vi "RT Loop - Log Data_1.vi"(7 "G1 trigger":bool, 8 "error in (no error)":errorcluster, 9 "Log File out":refnum<k34>, 10 "Array":waveform(dbl)[](array[waveform]), 11 "Message Queue":refnum<queue>) -> ()   [LabVIEW 2017]
doc: "Receive triggered data from Analyze Acceleration Loop and log the data to disk."
uses:
  Globals/Global - All RT Loop Stop.vi
  UI Error Handlers/support/Message Queue/Message Cluster.ctl
  UI Error Handlers/support/Message Queue/Message Queue.lvlib
panel:
  out "AVI Path":path
  out "Acceleration Log Folder":path=path "/home/lvuser/Log/logfiles_deploy"
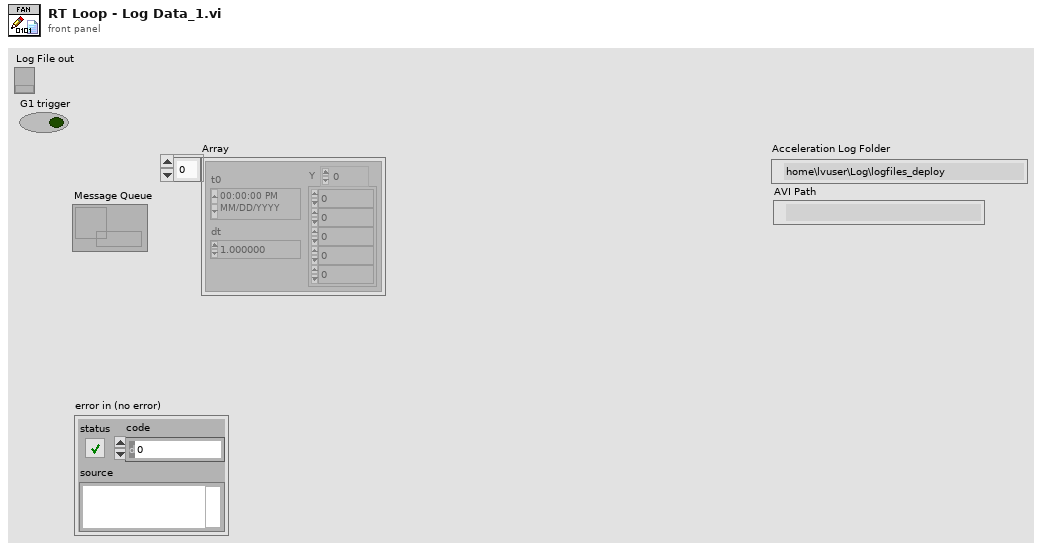
[diagram p1: front panel]
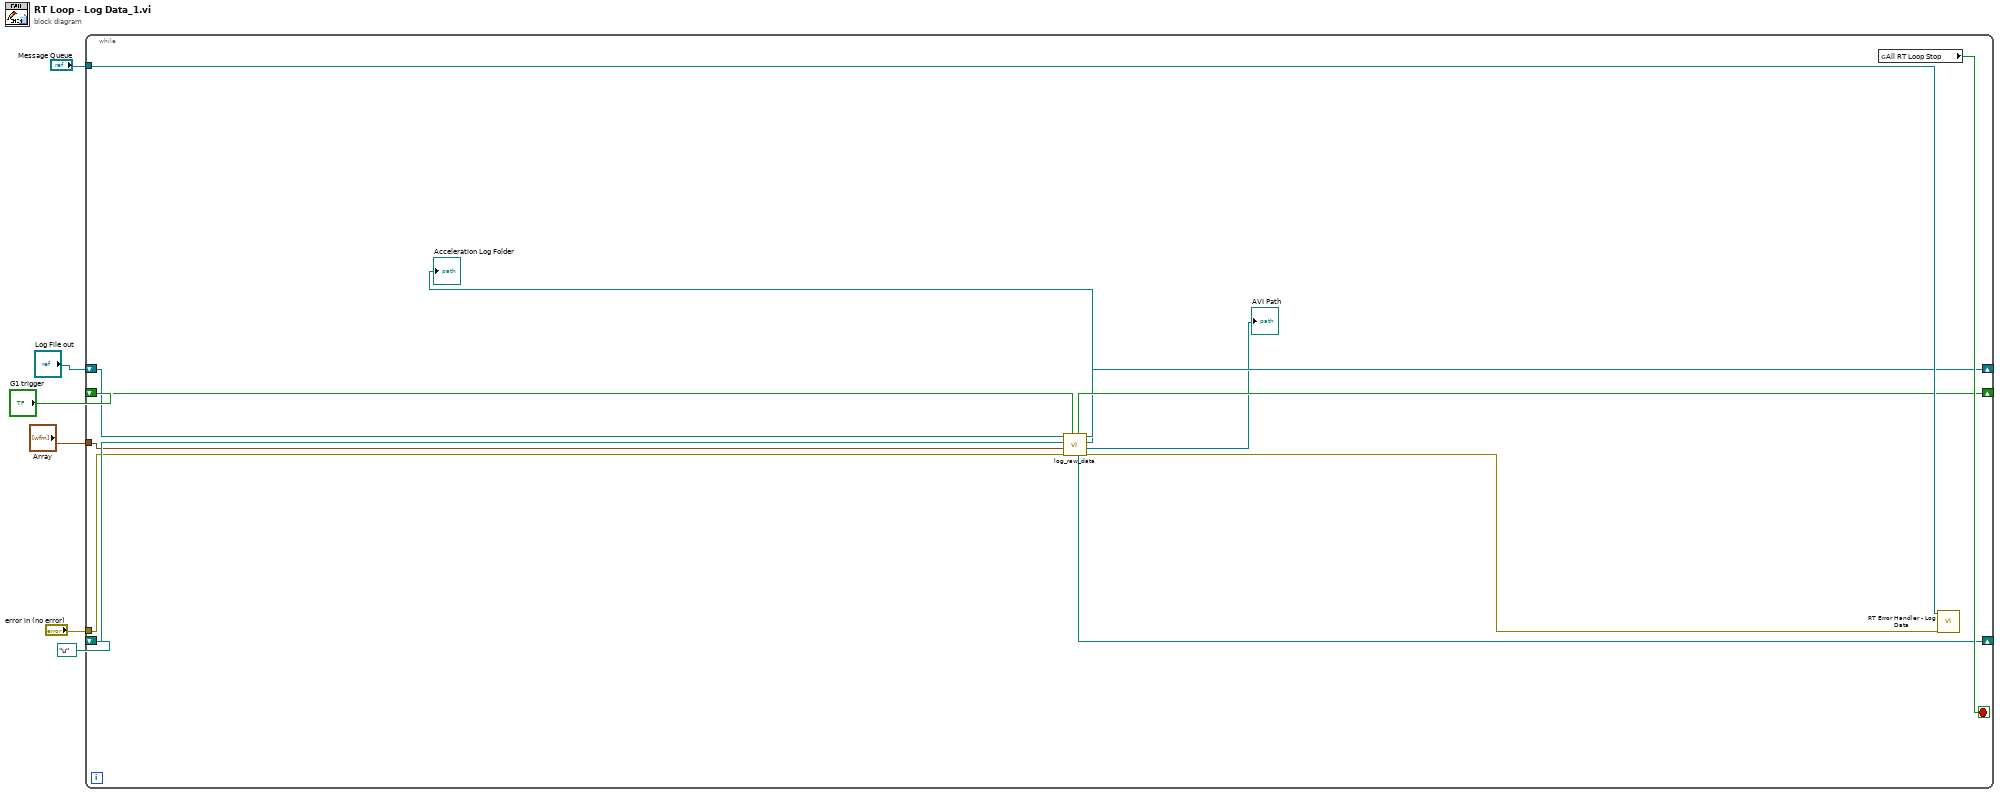
[diagram p0: block diagram]
diagram:
  n1 = while {
    tunnel: "Message Queue" -> [w18]
    tunnel: "error in (no error)" -> [w9]
    shift-right: [w16] -> _
    shift-left: path "u:/" ("AVI Path") -> [w15]
    shift-right: [w14] -> _
    shift-left: "G1 trigger" -> [w13]
    shift-right: [w12] -> _
    shift-left: "Log File out" -> [w11]
    tunnel: "Array" -> [w10]
    stop <- w19 stop-if-true
    n2 = call "log_raw_data.vi"("G1 trigger in"=w13, "error in (no error)"=w9, "Array"=w10, "AVI Path in"=w15, "Refnum in"=w11) -> ("error out"=w17:errorcluster, "AVI Path out"=→"AVI Path":path, "Acceleration Log Folder"=→"Acceleration Log Folder":path, "Refnum out"=w12:refnum<k34>, "AVI Path 3"=w16:path, "G1 trigger out"=w14:bool)  [unwired: 1 in]
    n3 = global read "Global - All RT Loop Stop.vi" "All RT Loop Stop"() -> (w19:bool)
    n4 = call "RT Error Handler - Log Data.vi"("error in (no error)"=w17, "Message Queue"=w18) -> ()  [unwired: 9 in, 1 out]
  }
